vi "Cartesian To Complex - RM,RM.vi"(1 "Real Matrix I":T1, 2 "Real Matrix R":T1) -> (0 "R + Ii":T2)   [LabVIEW 2020, in "NI_Matrix.lvlib"]
doc: "Creates a complex number from two values in rectangular notation."
uses:
  <vilib>/Analysis/Matrix/NI_Matrix.lvlib
  <vilib>/Analysis/Matrix/Datatypes/RealMatrix.ctl
  <vilib>/Analysis/Matrix/Datatypes/ComplexMatrix.ctl
  <vilib>/Analysis/Matrix/Numeric/Conversions/Matrix To Array - RM.vi
  <vilib>/Analysis/Matrix/Numeric/Conversions/Array To Matrix - CA2.vi
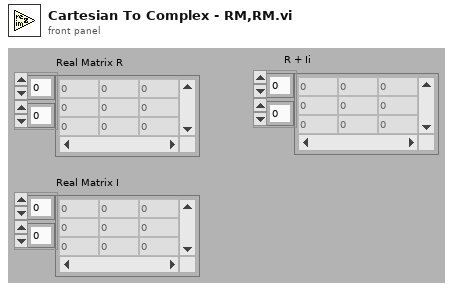
[diagram p1: front panel]
types:
  T1 = typedef "NI_Matrix.lvlib/RealMatrix.ctl" = dbl[][]
  T2 = typedef "NI_Matrix.lvlib/ComplexMatrix.ctl" = cdb[][]
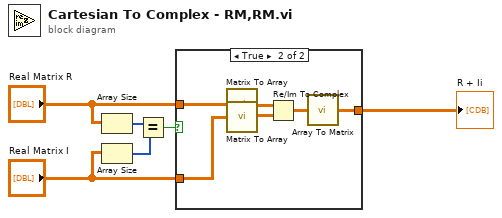
[diagram p0: block diagram]
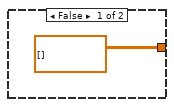
[diagram p2: hidden frame]
diagram:
  n1 = Array Size(array="Real Matrix R") -> (size(s)=w4:i32[])
  n2 = Array Size(array="Real Matrix I") -> (size(s)=w5:i32[])
  n3 = Equal?(x=w4, y=w5) -> (x = y?=w1:bool)
  n4 = case shown="True" w1 {
    tunnel: "Real Matrix R" -> [_ w10]
    tunnel: "Real Matrix I" -> [_ w11]
    tunnel: [T2 [] ("R + Ii") w8] -> w6
    frame False {
    }
    frame True {
      n5 = call-poly <vilib>:"Matrix To Array.vi"("Real Matrix"=w10) -> ("Real 2D Array"=w12:dbl[][])
      n6 = call-poly <vilib>:"Matrix To Array.vi"("Real Matrix"=w11) -> ("Real 2D Array"=w13:dbl[][])
      n7 = Re/Im To Complex(1:w13, 2:w12) -> (0:w9:cdb[][])
      n8 = call-poly <vilib>:"Array To Matrix.vi"("Complex 2D Array"=w9) -> ("Complex Matrix"=w8:T2)
    }
  }
  "R + Ii" <- w6
